vi "write coils.vi"(6 "Ignore Mask?":bool, 7 "Write Mask":bool[](array[boolean]), 8 "error in (no error)":errorcluster, 9 "Channel Data":T1[](array[typedef]), 10 "Values":dbl[](array[numeric]), 11 "Modbus API.lvlibp:Modbus API":refnum<class "Modbus API.lvclass">) -> (0 "error out":errorcluster)   [LabVIEW 2020, in "Modbus Master Engine.lvlib"]
uses:
  Modbus Master Engine.lvlib
  Shared/Controls/Data Model/Channel.ctl
  System Explorer/SubVIs/Modbus Type.ctl
  <vilib>/NI VeriStand/Custom Device API/Custom Device Channel Type.ctl
  Shared/Controls/Data Model/Mapping.ctl
  Shared/Controls/Data Model/DataType.ctl
  <vilib>/NI VeriStand/Custom Device API/Custom Device Item Ref.ctl
  Modbus API.lvlibp/API/Modbus API.lvclass
  Shared/Modbus Master Shared.lvlib
  <vilib>/NI VeriStand/Custom Device API/Custom Device API.lvlib
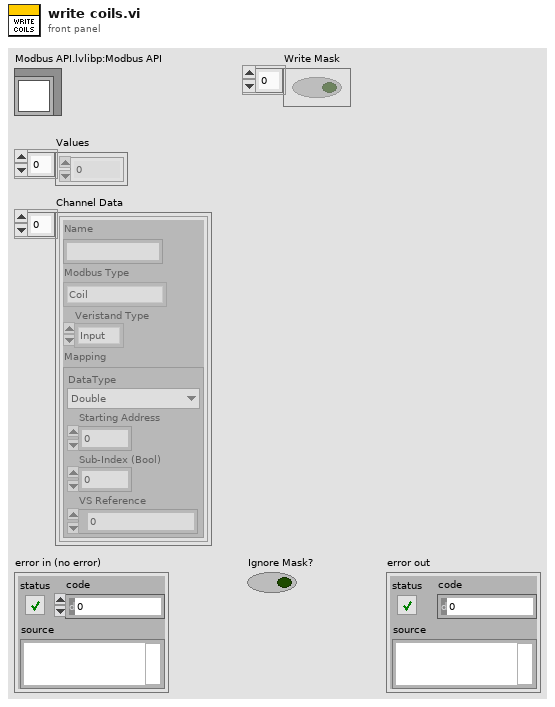
[diagram p1: front panel]
types:
  T1 = typedef "Modbus Master Shared.lvlib/Channel.ctl" = cluster{"Name":string, "Modbus Type":T2, "Veristand Type":T3, "Mapping":T4}
  T2 = typedef "Modbus Master Shared.lvlib/Modbus Type.ctl" = enum16{"Coil", "Discrete Input", "Holding Register", "Input Register"}
  T3 = typedef "Custom Device API.lvlib/Custom Device Channel Type.ctl" = enum16{"Input", "Output"}
  T4 = typedef "Modbus Master Shared.lvlib/Mapping.ctl" = cluster{"DataType":T5, "Starting Address":u16, "Sub-Index (Bool)":u16, "VS Reference":T6}
  T5 = typedef "Modbus Master Shared.lvlib/DataType.ctl" = enum16{"Double", "Single", "I64", "I32", "I16", "I8", "U64", "U32", "U16", "U8", "Boolean"}
  T6 = typedef "Custom Device API.lvlib/Custom Device Item Ref.ctl" = u64
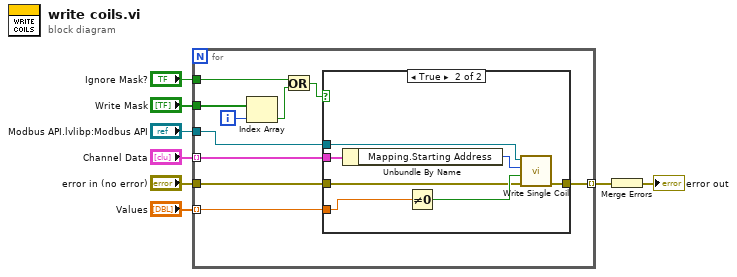
[diagram p0: block diagram]
diagram:
  n1 = for {
    tunnel: "Modbus API.lvlibp:Modbus API" -> [w18]
    tunnel: "Values" -> [w16] mode=indexing
    tunnel: "Write Mask" -> [w11]
    tunnel: "Channel Data" -> [w15] mode=indexing
    tunnel: "Ignore Mask?" -> [w13]
    tunnel: "error in (no error)" -> [w17]
    tunnel: [w14] -> w2 mode=indexing
    i -> [w10]
    n2 = Index Array(array=w11, index=w10) -> (element=w9:bool)
    n3 = Or(x=w13, y=w9) -> (x .or. y?=w12:bool)
    n4 = case shown="True" w12 {
      tunnel: w18 -> [_ w21]
      tunnel: w17 -> [w19 w22]
      tunnel: [w19 w20] -> w14
      tunnel: w16 -> [_ w26]
      tunnel: w15 -> [_ w25]
      frame False {
      }
      frame True {
        n5 = Unbundle By Name(w25) -> ("Mapping.Starting Address"=w24:u16)
        n6 = Not Equal To 0?(x=w26) -> (x != 0?=w23:bool)
        n7 = call-dynamic "Write Single Coil.vi"("error in"=w22, "coil to write"=w23, "address"=w24, "Modbus instance in"=w21) -> ("error out"=w20:errorcluster)  [unwired: 6 in, 1 out]
      }
    }
  }
  n8 = Merge Errors(w2) -> (→"error out":errorcluster)
